vi "Get Mercurial Changeset.vi"(9 "not found string (\"\")":string, 11 "Path":path) -> (1 "Change Set String":string, 2 "changeset hash number":u64 format="%x", 3 "changeset rev":i32, 4 "repo error?":bool)   [LabVIEW 2017]
doc: "Returns the current SVN revision and latest available SVN revision of the inputed vi or directory. Returns -1 if not versioned in SVN."
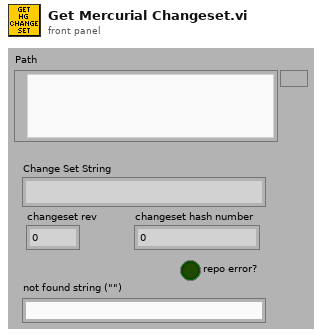
[diagram p1: front panel]
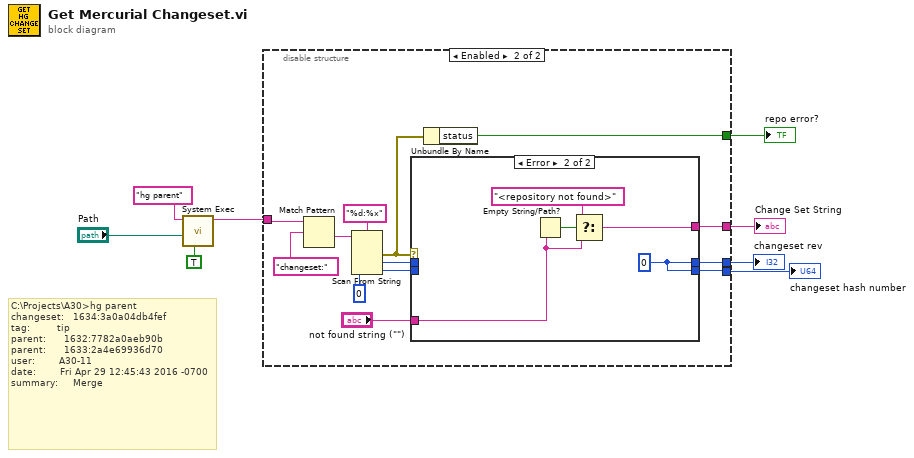
[diagram p0: block diagram]
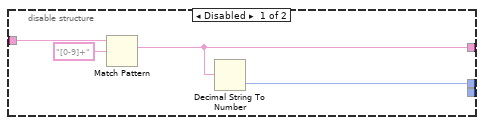
[diagram p2: hidden frame]
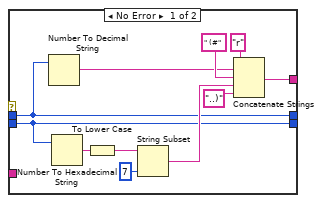
[diagram p3: hidden frame]
diagram:
  # "C:\\Projects\\A30>hg parent\nchangeset:   1634:3a0a04db4fef\ntag:         tip\nparent:      1632:7782a0aeb90b\nparent:      1633:2a4e69936d70\nuser:        A30-11\ndate:        Fri Apr 29 12:45:43 2016 -0700\nsummary:     Merge"
  n1 = call <vilib>:"System Exec.vi"("run minimized? (F)"=TRUE, "working directory"="Path", "command line"="hg parent") -> ("standard output"=w5:string)  [unwired: 5 in, 3 out]
  n2 = disable-structure shown="Enabled" {
    disable-tunnel: w5 -> [w12 w25]
    disable-tunnel: [w10 w18] -> w4
    disable-tunnel: [w9 w17] -> w3
    disable-tunnel: [_ w16] -> w2
    disable-tunnel: [_ w13] -> w1
    frame Disabled {
      n3 = Match Pattern(string=w12, regular expression="[0-9]+") -> (match substring=w10:string)  [unwired: 1 in, 3 out]
      n4 = Decimal String To Number(string=w10) -> (number=w9:i32)  [unwired: 2 in, 1 out]
    }
    frame Enabled {
      n5 = Match Pattern(string=w25, regular expression="changeset:") -> (after substring=w23:string)  [unwired: 1 in, 3 out]
      n6 = Scan From String(format string="%d:%x", input string=w23, default 2=u64 0) -> (error out=w14:errorcluster, output 1=w21:i32, output 2=w20:u64)  [unwired: 3 in, 2 out]
      n7 = case shown="Error" w14 {
        tunnel: w21 -> [w27 _]
        tunnel: w20 -> [w26 _]
        tunnel: [w28 w38] -> w18
        tunnel: [w27 w41] -> w17
        tunnel: [w26 w41] -> w16
        tunnel: "not found string (\"\")" -> [_ w37]
        frame No Error {
          n8 = Number To Decimal String(number=w27) -> (decimal integer string=w30:string)  [unwired: 1 in]
          n9 = Number To Hexadecimal String(2:w26) -> (0:w36:string)  [unwired: 1 in]
          n10 = To Lower Case(string=w36) -> (all lower case string=w35:string)
          n11 = String Subset(string=w35, length (rest)=7 ("offset (0)")) -> (substring=w29:string)  [unwired: 1 in]
          n12 = Concatenate Strings("r" ("string"), w30, " (#", w29, "..)") -> (w28:string)
        }
        frame Error {
          w41 = 0
          n13 = Empty String/Path?(string/path=w37) -> (empty?=w40:bool)
          n14 = Select(t="<repository not found>", s=w40, f=w37) -> (s? t:f=w38:string)
        }
      }
      n15 = Unbundle By Name(w14) -> ("status"=w13:bool)
    }
  }
  "Change Set String" <- w4
  "changeset rev" <- w3
  "changeset hash number" <- w2
  "repo error?" <- w1
